vi "Stop.vi"(1 "Stop?":bool) -> (0 "Stop Called":bool)   [LabVIEW 2013]
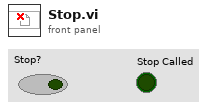
[diagram p1: front panel]
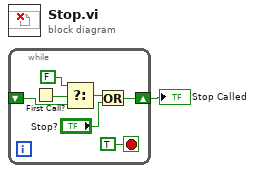
[diagram p0: block diagram]
diagram:
  n1 = while {
    shift-right: [w3] -> w1
    shift-left: _ -> [w6]
    stop <- TRUE stop-if-true
    n2 = First Call?() -> (First Call?: T/F=w8:bool)
    n3 = Select(t=FALSE, s=w8, f=w6) -> (s? t:f=w5:bool)
    n4 = Or(x=w5, y="Stop?") -> (x .or. y?=w3:bool)
  }
  "Stop Called" <- w1
